vi "Obtain Message Queue.vi"(8 "error in (no error)":T1 caption="Fehler (Eingang, kein Fehler)") -> (0 "error out":T1 caption="Fehler (Ausgang)", 3 "Nachrichten-Queue":refnum<queue>)   [LabVIEW 2014, in "MyQH Message Queue.lvlib"]
doc: "Erstellt eine Queue mit dem Datentyp \"Nachrichten-Cluster\"."
uses:
  MyQH Message Queue.lvlib
  Message Cluster.ctl
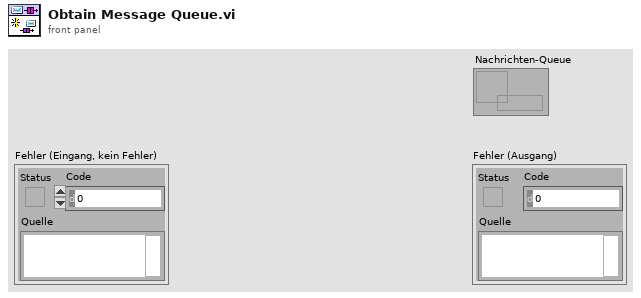
[diagram p1: front panel]
types:
  T1 = cluster{"Status":bool, "Code":i32, "Quelle":string}
  T2 = typedef "MyQH Message Queue.lvlib/Message Cluster.ctl" = cluster{"Nachricht":string, "Nachrichtendaten":variant}
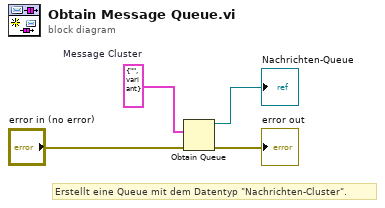
[diagram p0: block diagram]
diagram:
  w4 = T2 {"Nachricht"="", "Nachrichtendaten"=variant}  # Message Cluster
  # "Erstellt eine Queue mit dem Datentyp \"Nachrichten-Cluster\"."
  n1 = Obtain Queue(element data type=w4, error in (no error)="error in (no error)") -> (queue out=→"Nachrichten-Queue":refnum<queue>, error out=→"error out":errorcluster)  [unwired: 3 in, 1 out]
